vi "movement control.vi"(0 "pos x":i16, 2 "lift":i16, 3 "current lift":i16, 5 "pos y":i16, 9 "current x 2":i16, 11 "current y 2":i16, 13 "gripper":i16, 14 "current gripper":i16) -> (4 "target x 2":i16, 6 "target y 2":i16, 10 "target lift":i16, 15 "target gripper":i16)   [LabVIEW 2014]
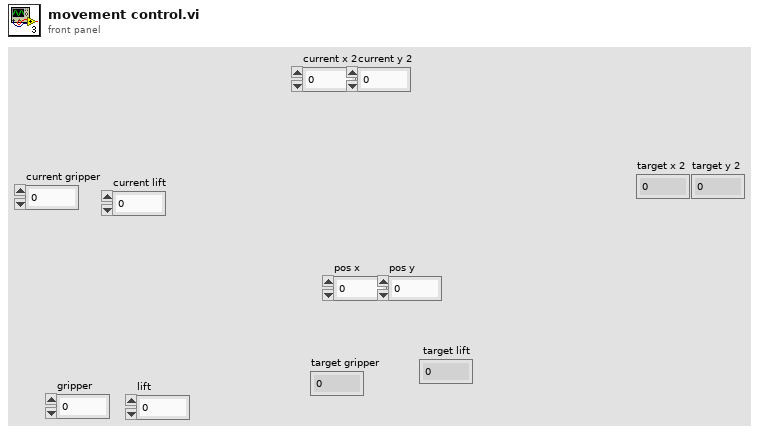
[diagram p1: front panel]
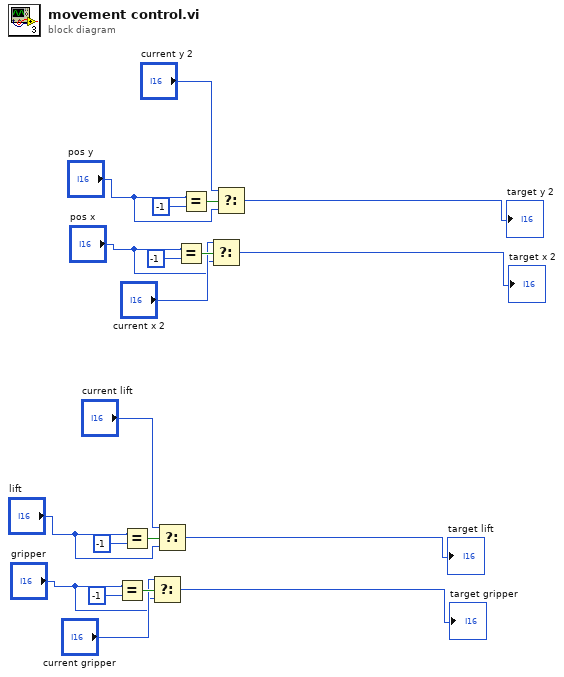
[diagram p0: block diagram]
diagram:
  n1 = Equal?(x="gripper", y=-1) -> (x = y?=w7:bool)
  n2 = Equal?(x="lift", y=-1) -> (x = y?=w9:bool)
  n3 = Select(t="current gripper", s=w7, f="gripper") -> (s? t:f=→"target gripper":i16)
  n4 = Select(t="current lift", s=w9, f="lift") -> (s? t:f=→"target lift":i16)
  n5 = Equal?(x="pos x", y=-1) -> (x = y?=w17:bool)
  n6 = Equal?(x="pos y", y=-1) -> (x = y?=w19:bool)
  n7 = Select(t="current x 2", s=w17, f="pos x") -> (s? t:f=→"target x 2":i16)
  n8 = Select(t="current y 2", s=w19, f="pos y") -> (s? t:f=→"target y 2":i16)
